vi "PXI-StopDAQ (short icon).vi"(0 "error in (no error)":errorcluster, 1 "Wait for DAQ to stop? (T)":bool=TRUE) -> (2 "error out":errorcluster)   [LabVIEW 2015]
doc: "Sets global variables that terminate the main DAQ loop."
uses:
  DAQ Engine VIs/PXI Globals.vi
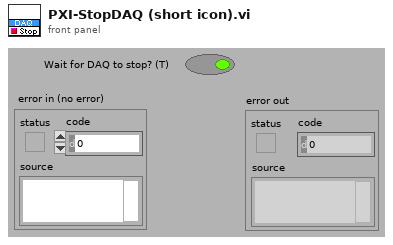
[diagram p1: front panel]
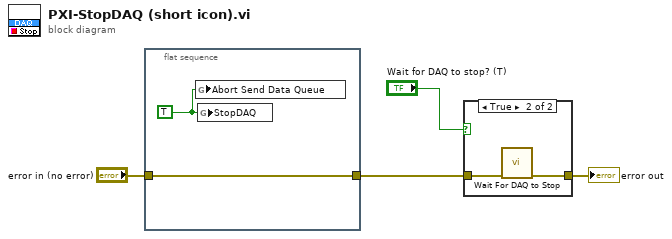
[diagram p0: block diagram]
diagram:
  n1 = flat-sequence {
    tunnel: "error in (no error)" -> [w5]
    tunnel: [w5] -> w3
    frame #0 {
      w6 = TRUE ("StopDAQ")
      n2 = global write "PXI Globals.vi" "Abort Send Data Queue"(w6) -> ()
      n3 = global write "PXI Globals.vi" "StopDAQ"(w6) -> ()
    }
  }
  n4 = case shown="True" "Wait for DAQ to stop? (T)" {
    tunnel: w3 -> [w7 w9]
    tunnel: [w7 w8] -> w1
    frame False {
    }
    frame True {
      n5 = call "Wait For DAQ to Stop.vi"("error in (no error)"=w9) -> ("error out"=w8:errorcluster)  [unwired: 10 in]
    }
  }
  "error out" <- w1
